vi "Register TypeMap.vi"(8 "error in (no error)":errorcluster, 10 "TypeMap in":refnum<class "TypeMap.lvclass">, 11 "object in":refnum<class>) -> (0 "error out":errorcluster, 2 "replaced?":bool, 3 "object out":refnum<class>)   [LabVIEW 2020, in "ORM.lvlib" / "TypeMap.lvclass"]
uses:
  TypeMap.lvclass
  TypeMap.lvclass/TypeMap.ctl
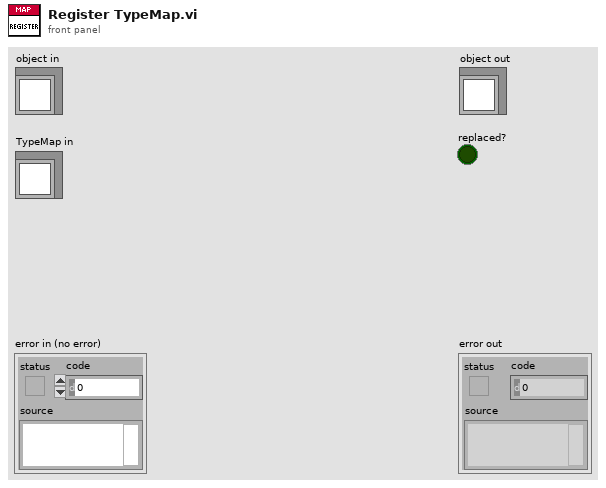
[diagram p1: front panel]
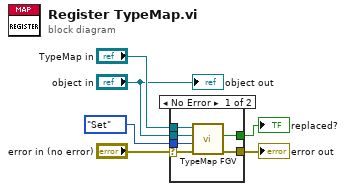
[diagram p0: block diagram]
diagram:
  n1 = case shown="No Error" "error in (no error)" {
    selector: "error in (no error)" -> [w9 w13]
    tunnel: "TypeMap in" -> [w12 _]
    tunnel: "object in" -> [w11 _]
    tunnel: enum16{"Get", "Set"}."Set" ("Action") -> [w10 _]
    tunnel: [w8 w13] -> w2
    tunnel: [w7 _] -> w1
    frame No Error {
      n2 = call "TypeMap FGV.vi"("error in (no error)"=w9, "Action"=w10, "object"=w11, "TypeMap in"=w12) -> ("error out"=w8:errorcluster, "found/replaced?"=w7:bool)  [unwired: 5 in, 1 out]
    }
    frame Error {
    }
  }
  "error out" <- w2
  "replaced?" <- w1
  "object out" <- "object in"
